vi "H036 Harsh Pandit SCADA Lab 4a Sem 6.vi"() -> ()   [LabVIEW 2018]
panel:
  out "Waveform Chart":dynamicdata(graph)
  in  "Frequency":dbl(knob) scale=0.0..5.0
  in  "Amplitude":dbl(knob) scale=0.0..20.0
  # "Experiment 4a: Develope sine wave generator using express VI vary the amplitude and frequency using knob"
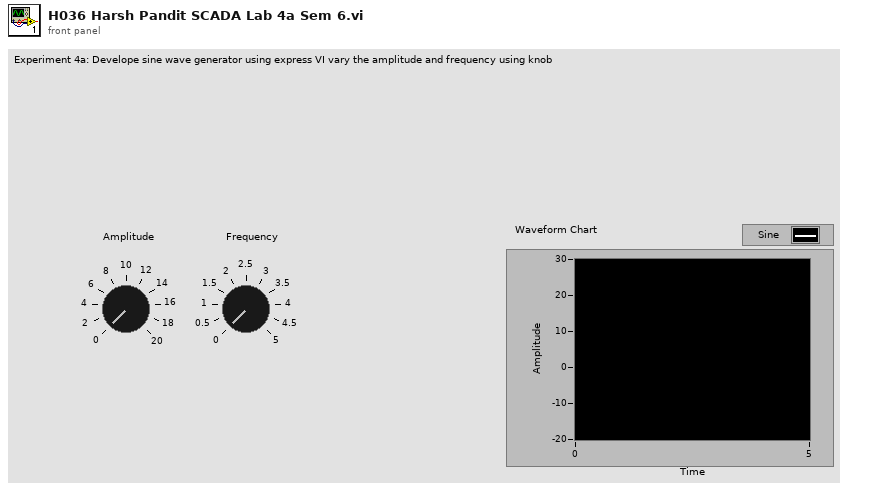
[diagram p1: front panel]
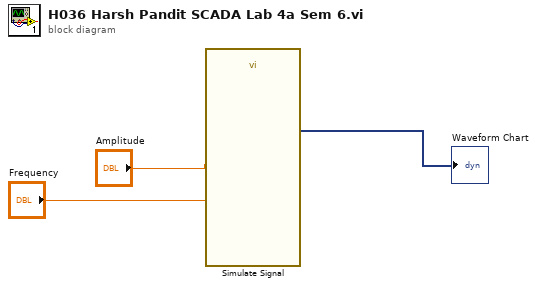
[diagram p0: block diagram]
diagram:
  n1 = call "Simulate Signal"("Frequency"="Frequency", "Amplitude"="Amplitude") -> ("Sine"=→"Waveform Chart":dynamicdata)  [unwired: 12 in, 1 out]
